vi "DisplayJson.vi"(11 "JSON String In":string="[{\"version\":\"1.0.0\",\"header\":{\"creationDate\":\"2022-06-03T00:00:00\",\"remarks\":\"\",\"serialNumber\":\"98172\",\"productNumber\":\"123021.1804\",\"productType\":\"PAA-9L\",\"pressureType\":2,\"productSeries\":\"9L\",\"compensatedTemperatureRange\":{\"min\":-10.0,\"max\":80.0,\"unit\":4},\"compensatedPressureRange\":{\"min\":0.0,\"max\":0.35,\"unit\":3},\"electricSupply\":{\"magnitude\":1.0,\"unit\":18},\"orderNumber\":9990266,\"orderPosition\":3,\"orderTargetDispatchDate\":\"2022-06-02T00:00:00+00:00\",\"customerName\":\"DemoData Inc.\",\"customerNumber\":12345678,\"customerOrderNumber\":\"Cust-9990266-123\",\"customerReferenceNumber\":\"\",\"customerProductT...") -> ()   [LabVIEW 2017] (continued)
\"unit\":4},\"error\":{\"magnitude\":0.10911646,\"unit\":4}}}}}},{\"reference\":\"F_12300_XX_0000098765\",\"environmentTarget\":{\"pressure\":{\"magnitude\":0.11,\"unit\":3},\"temperature\":{\"magnitude\":80.0,\"unit\":4}},\"environment\":{\"pressure\":{\"magnitude\":0.11,\"unit\":3},\"temperature\":{\"magnitude\":79.9513,\"unit\":4},\"supply\":{\"magnitude\":1.0,\"unit\":18}},\"raw\":{\"signal\":{\"magnitude\":34.075381003,\"unit\":22},\"bridgeResistance\":{\"magnitude\":4098.6572078,\"unit\":28}},\"compensated\":{\"mathematicalModels\":{\"MM0123\":{\"pressure\":{\"output\":{\"magnitude\":0.10996,\"unit\":3},\"error\":{\"magnitude\":-0.011442623,\"unit\":7}},\"temperature\":{\"output\":{\"magnitude\":80.0644,\"unit\":4},\"error\":{\"magnitude\":0.11306469,\"unit\":4}}}}}},{\"reference\":\"F_12300_XX_0000098765\",\"environmentTarget\":{\"pressure\":{\"magnitude\":0.19,\"unit\":3},\"temperature\":{\"magnitude\":80.0,\"unit\":4}},\"environment\":{\"pressure\":{\"magnitude\":0.189999,\"unit\":3},\"temperature\":{\"magnitude\":79.9513,\"unit\":4},\"supply\":{\"magnitude\":1.0,\"unit\":18}},\"raw\":{\"signal\":{\"magnitude\":46.277899936,\"unit\":22},\"bridgeResistance\":{\"magnitude\":4094.0695855,\"unit\":28}},\"compensated\":{\"mathematicalModels\":{\"MM0123\":{\"pressure\":{\"output\":{\"magnitude\":0.190002,\"unit\":3},\"error\":{\"magnitude\":0.00090359414,\"unit\":7}},\"temperature\":{\"output\":{\"magnitude\":80.0722,\"unit\":4},\"error\":{\"magnitude\":0.12084368,\"unit\":4}}}}}},{\"reference\":\"F_12300_XX_0000098765\",\"environmentTarget\":{\"pressure\":{\"magnitude\":0.27,\"unit\":3},\"temperature\":{\"magnitude\":80.0,\"unit\":4}},\"environment\":{\"pressure\":{\"magnitude\":0.27,\"unit\":3},\"temperature\":{\"magnitude\":79.9513,\"unit\":4},\"supply\":{\"magnitude\":1.0,\"unit\":18}},\"raw\":{\"signal\":{\"magnitude\":58.449048989,\"unit\":22},\"bridgeResistance\":{\"magnitude\":4089.5073863,\"unit\":28}},\"compensated\":{\"mathematicalModels\":{\"MM0123\":{\"pressure\":{\"output\":{\"magnitude\":0.270033,\"unit\":3},\"error\":{\"magnitude\":0.0095410356,\"unit\":7}},\"temperature\":{\"output\":{\"magnitude\":80.0777,\"unit\":4},\"error\":{\"magnitude\":0.12631932,\"unit\":4}}}}}},{\"reference\":\"F_12300_XX_0000098765\",\"environmentTarget\":{\"pressure\":{\"magnitude\":0.35,\"unit\":3},\"temperature\":{\"magnitude\":80.0,\"unit\":4}},\"environment\":{\"pressure\":{\"magnitude\":0.349991,\"unit\":3},\"temperature\":{\"magnitude\":79.9513,\"unit\":4},\"supply\":{\"magnitude\":1.0,\"unit\":18}},\"raw\":{\"signal\":{\"magnitude\":70.576898184,\"unit\":22},\"bridgeResistance\":{\"magnitude\":4085.0103843,\"unit\":28}},\"compensated\":{\"mathematicalModels\":{\"MM0123\":{\"pressure\":{\"output\":{\"magnitude\":0.349975,\"unit\":3},\"error\":{\"magnitude\":-0.0045630258,\"unit\":7}},\"temperature\":{\"output\":{\"magnitude\":80.084,\"unit\":4},\"error\":{\"magnitude\":0.13265707,\"unit\":4}}}}}}]},{\"version\":\"1.0.0\",\"header\":{\"creationDate\":\"2022-06-03T00:00:00\",\"remarks\":\"\",\"serialNumber\":\"98120\",\"productNumber\":\"123021.1804\",\"productType\":\"PAA-9L\",\"pressureType\":2,\"productSeries\":\"9L\",\"compensatedTemperatureRange\":{\"min\":-10.0,\"max\":80.0,\"unit\":4},\"compensatedPressureRange\":{\"min\":0.0,\"max\":0.35,\"unit\":3},\"electricSupply\":{\"magnitude\":1.0,\"unit\":18},\"orderNumber\":9990266,\"orderPosition\":3,\"orderTargetDispatchDate\":\"2022-06-02T00:00:00+00:00\",\"customerName\":\"DemoData Inc.\",\"customerNumber\":12345678,\"customerOrderNumber\":\"Cust-9990266-123\",\"customerReferenceNumber\":\"\",\"customerProductType\":\"123021-1804 Rev.AA\"},\"compensationMethods\":{\"mathematicalModels\":{\"MM0123\":{\"modelType\":\"MM0123\",\"productNumber\":\"000000.0000\",\"compensatedTemperatureRange\":{\"min\":-10.0,\"max\":80.0,\"unit\":4},\"compensatedPressureRange\":{\"min\":0.0,\"max\":0.35,\"unit\":3},\"electricSupply\":{\"magnitude\":1.0,\"unit\":18},\"parts\":{\"pressure\":{\"inputs\":[\"Sig\",\"R\"],\"output\":\"P\",\"description\":\"P = f(Sig,R)\",\"coefficients\":[[3.80687640842,-0.00383024726793,1.42827172301E-06,-2.38902903502E-10,1.49525310822E-14],[-0.0978417022725,0.000104324759416,-3.89249748451E-08,6.44275711238E-12,-4.00281485262E-16],[-0.000392661762146,4.52316475722E-07,-1.9265072904E-10,3.61496115335E-14,-2.52797959852E-18]]},\"temperature\":{\"inputs\":[\"R\",\"Sig\"],\"output\":\"T\",\"description\":\"T = f(R,Sig)\",\"coefficients\":[[-7952.96201197,-2.02662210439,0.0134421000875],[7.80033862746,0.00330646246975,-1.59232351911E-05],[-0.00293461659049,-1.72390715848E-06,6.89820469355E-09],[5.0021540696E-07,3.72029008192E-10,-1.30570761964E-12],[-3.21770300206E-11,-2.89606535877E-14,9.15121335916E-17]]}}}}},\"measurements\":[{\"reference\":\"F_12300_XX_0000098765\",\"environmentTarget\":{\"pressure\":{\"magnitude\":0.03,\"unit\":3},\"temperature\":{\"magnitude\":-10.0,\"unit\":4}},\"environment\":{\"pressure\":{\"magnitude\":0.0300016,\"unit\":3},\"temperature\":{\"magnitude\":-10.7286,\"unit\":4},\"supply\":{\"magnitude\":1.0,\"unit\":18}},\"raw\":{\"signal\":{\"magnitude\":17.647568183,\"unit\":22},\"bridgeResistance\":{\"magnitude\":3284.2199645,\"unit\":28}},\"compensated\":{\"mathematicalModels\":{\"MM0123\":{\"pressure\":{\"output\":{\"magnitude\":0.0300151,\"unit\":3},\"error\":{\"magnitude\":0.0038534803,\"unit\":7}},\"temperature\":{\"output\":{\"magnitude\":-10.8543,\"unit\":4},\"error\":{\"magnitude\":-0.12565537,\"unit\":4}}}}}},{\"reference\":\"F_12300_XX_0000098765\",\"environmentTarget\":{\"pressure\":{\"magnitude\":0.11,\"unit\":3},\"temperature\":{\"magnitude\":-10.0,\"unit\":4}},\"environment\":{\"pressure\":{\"magnitude\":0.109994,\"unit\":3},\"temperature\":{\"magnitude\":-10.7286,\"unit\":4},\"supply\":{\"magnitude\":1.0,\"unit\":18}},\"raw\":{\"signal\":{\"magnitude\":29.623305989,\"unit\":22},\"bridgeResistance\":{\"magnitude\":3279.6852656,\"unit\":28}},\"compensated\":{\"mathematicalModels\":{\"MM0123\":{\"pressure\":{\"output\":{\"magnitude\":0.10996,\"unit\":3},\"error\":{\"magnitude\":-0.0096543576,\"unit\":7}},\"temperature\":{\"output\":{\"magnitude\":-10.8536,\"unit\":4},\"error\":{\"magnitude\":-0.12492151,\"unit\":4}}}}}},{\"reference\":\"F_12300_XX_0000098765\",\"environmentTarget\":{\"pressure\":{\"magnitude\":0.19,\"unit\":3},\"temperature\":{\"magnitude\":-10.0,\"unit\":4}},\"environment\":{\"pressure\":{\"magnitude\":0.190007,\"unit\":3},\"temperature\":{\"magnitude\":-10.7286,\"unit\":4},\"supply\":{\"magnitude\":1.0,\"unit\":18}},\"raw\":{\"signal\":{\"magnitude\":41.5629955,\"unit\":22},\"bridgeResistance\":{\"magnitude\":3275.2173858,\"unit\":28}},\"compensated\":{\"mathematicalModels\":{\"MM0123\":{\"pressure\":{\"output\":{\"magnitude\":0.190015,\"unit\":3},\"error\":{\"magnitude\":0.0022835569,\"unit\":7}},\"temperature\":{\"output\":{\"magnitude\":-10.8576,\"unit\":4},\"error\":{\"magnitude\":-0.12895315,\"unit\":4}}}}}},{\"reference\":\"F_12300_XX_0000098765\",\"environmentTarget\":{\"pressure\":{\"magnitude\":0.27,\"unit\":3},\"temperature\":{\"magnitude\":-10.0,\"unit\":4}},\"environment\":{\"pressure\":{\"magnitude\":0.270011,\"unit\":3},\"temperature\":{\"magnitude\":-10.7286,\"unit\":4},\"supply\":{\"magnitude\":1.0,\"unit\":18}},\"raw\":{\"signal\":{\"magnitude\":53.446990918,\"unit\":22},\"bridgeResistance\":{\"magnitude\":3270.9221092,\"unit\":28}},\"compensated\":{\"mathematicalModels\":{\"MM0123\":{\"pressure\":{\"output\":{\"magnitude\":0.270044,\"unit\":3},\"error\":{\"magnitude\":0.0095289216,\"unit\":7}},\"temperature\":{\"output\":{\"magnitude\":-10.8518,\"unit\":4},\"error\":{\"magnitude\":-0.12313925,\"unit\":4}}}}}},{\"reference\":\"F_12300_XX_0000098765\",\"environmentTarget\":{\"pressure\":{\"magnitude\":0.35,\"unit\":3},\"temperature\":{\"magnitude\":-10.0,\"unit\":4}},\"environment\":{\"pressure\":{\"magnitude\":0.350004,\"unit\":3},\"temperature\":{\"magnitude\":-10.7286,\"unit\":4},\"supply\":{\"magnitude\":1.0,\"unit\":18}},\"raw\":{\"signal\":{\"magnitude\":65.267069587,\"unit\":22},\"bridgeResistance\":{\"magnitude\":3266.656716,\"unit\":28}},\"compensated\":{\"mathematicalModels\":{\"MM0123\":{\"pressure\":{\"output\":{\"magnitude\":0.349998,\"unit\":3},\"error\":{\"magnitude\":-0.0016541156,\"unit\":7}},\"temperature\":{\"output\":{\"magnitude\":-10.8581,\"unit\":4},\"error\":{\"magnitude\":-0.12948393,\"unit\":4}}}}}},{\"reference\":\"F_12300_XX_0000098765\",\"environmentTarget\":{\"pressure\":{\"magnitude\":0.03,\"unit\":3},\"temperature\":{\"magnitude\":0.0,\"unit\":4}},\"environment\":{\"pressure\":{\"magnitude\":0.0300081,\"unit\":3},\"temperature\":{\"magnitude\":-0.629962,\"unit\":4},\"supply\":{\"magnitude\":1.0,\"unit\":18}},\"raw\":{\"signal\":{\"magnitude\":18.166060326,\"unit\":22},\"bridgeResistance\":{\"magnitude\":3353.9752499,\"unit\":28}},\"compensated\":{\"mathematicalModels\":{\"MM0123\":{\"pressure\":{\"output\":{\"magnitude\":0.030027,\"unit\":3},\"error\":{\"magnitude\":0.0053956345,\"unit\":7}},\"temperature\":{\"output\":{\"magnitude\":-0.756227,\"unit\":4},\"error\":{\"magnitude\":-0.12626536,\"unit\":4}}}}}},{\"reference\":\"F_12300_XX_0000098765\",\"environmentTarget\":{\"pressure\":{\"magnitude\":0.11,\"unit\":3},\"temperature\":{\"magnitude\":0.0,\"unit\":4}},\"environment\":{\"pressure\":{\"magnitude\":0.110003,\"unit\":3},\"temperature\":{\"magnitude\":-0.629962,\"unit\":4},\"supply\":{\"magnitude\":1.0,\"unit\":18}},\"raw\":{\"signal\":{\"magnitude\":30.109259393,\"unit\":22},\"bridgeResistance\":{\"magnitude\":3349.3967264,\"unit\":28}},\"compensated\":{\"mathematicalModels\":{\"MM0123\":{\"pressure\":{\"output\":{\"magnitude\":0.109974,\"unit\":3},\"error\":{\"magnitude\":-0.0081737866,\"unit\":7}},\"temperature\":{\"output\":{\"magnitude\":-0.762387,\"unit\":4},\"error\":{\"magnitude\":-0.13242561,\"unit\":4}}}}}},{\"reference\":\"F_12300_XX_0000098765\",\"environmentTarget\":{\"pressure\":{\"magnitude\":0.19,\"unit\":3},\"temperature\":{\"magnitude\":0.0,\"unit\":4}},\"environment\":{\"pressure\":{\"magnitude\":0.19,\"unit\":3},\"temperature\":{\"magnitude\":-0.629962,\"unit\":4},\"supply\":{\"magnitude\":1.0,\"unit\":18}},\"raw\":{\"signal\":{\"magnitude\":42.013989643,\"unit\":22},\"bridgeResistance\":{\"magnitude\":3344.9475418,\"unit\":28}},\"compensated\":{\"mathematicalModels\":{\"MM0123\":{\"pressure\":{\"output\":{\"magnitude\":0.189997,\"unit\":3},\"error\":{\"magnitude\":-0.00074399073,\"unit\":7}},\"temperature\":{\"output\":{\"magnitude\":-0.763716,\"unit\":4},\"error\":{\"magnitude\":-0.13375452,\"unit\":4}}}}}},{\"reference\":\"F_12300_XX_0000098765\",\"environmentTarget\":{\"pressure\":{\"magnitude\":0.27,\"unit\":3},\"temperature\":{\"magnitude\":0.0,\"unit\":4}},\"environment\":{\"pressure\":{\"magnitude\":0.270002,\"unit\":3},\"temperature\":{\"magnitude\":-0.629962,\"unit\":4},\"supply\":{\"magnitude\":1.0,\"unit\":18}},\"raw\":{\"signal\":{\"magnitude\":53.868228434,\"unit\":22},\"bridgeResistance\":{\"magnitude\":3340.5943615,\"unit\":28}},\"compensated\":{\"mathematicalModels\":{\"MM0123\":{\"pressure\":{\"output\":{\"magnitude\":0.270018,\"unit\":3},\"error\":{\"magnitude\":0.004524908,\"unit\":7}},\"temperature\":{\"output\":{\"magnitude\":-0.765646,\"unit\":4},\"error\":{\"magnitude\":-0.1356837,\"unit\":4}}}}}},{\"reference\":\"F_12300_XX_0000098765\",\"environmentTarget\":{\"pressure\":{\"magnitude\":0.35,\"unit\":3},\"temperature\":{\"magnitude\":0.0,\"unit\":4}},\"environment\":{\"pressure\":{\"magnitude\":0.349999,\"unit\":3},\"temperature\":{\"magnitude\":-0.629962,\"unit\":4},\"supply\":{\"magnitude\":1.0,\"unit\":18}},\"raw\":{\"signal\":{\"magnitude\":65.662121594,\"unit\":22},\"bridgeResistance\":{\"magnitude\":3336.3273067,\"unit\":28}},\"compensated\":{\"mathematicalModels\":{\"MM0123\":{\"pressure\":{\"output\":{\"magnitude\":0.349969,\"unit\":3},\"error\":{\"magnitude\":-0.0084390485,\"unit\":7}},\"temperature\":{\"output\":{\"magnitude\":-0.770185,\"unit\":4},\"error\":{\"magnitude\":-0.14022289,\"unit\":4}}}}}},{\"reference\":\"F_12300_XX_0000098765\",\"environmentTarget\":{\"pressure\":{\"magnitude\":0.03,\"unit\":3},\"temperature\":{\"magnitude\":20.0,\"unit\":4}},\"environment\":{\"pressure\":{\"magnitude\":0.0300042,\"unit\":3},\"temperature\":{\"magnitude\":19.5509,\"unit\":4},\"supply\":{\"magnitude\":1.0,\"unit\":18}},\"raw\":{\"signal\":{\"magnitude\":19.250087303,\"unit\":22},\"bridgeResistance\":{\"magnitude\":3510.6414258,\"unit\":28}},\"compensated\":{\"mathematicalModels\":{\"MM0123\":{\"pressure\":{\"output\":{\"magnitude\":0.0300123,\"unit\":3},\"error\":{\"magnitude\":0.0023081439,\"unit\":7}},\"temperature\":{\"output\":{\"magnitude\":19.5418,\"unit\":4},\"error\":{\"magnitude\":-0.0090331179,\"unit\":4}}}}}},{\"reference\":\"F_12300_XX_0000098765\",\"environmentTarget\":{\"pressure\":{\"magnitude\":0.11,\"unit\":3},\"temperature\":{\"magnitude\":20.0,\"unit\":4}},\"environment\":{\"pressure\":{\"magnitude\":0.109998,\"unit\":3},\"temperature\":{\"magnitude\":19.5509,\"unit\":4},\"supply\":{\"magnitude\":1.0,\"unit\":18}},\"raw\":{\"signal\":{\"magnitude\":31.186444983,\"unit\":22},\"bridgeResistance\":{\"magnitude\":3506.082338,\"unit\":28}},\"compensated\":{\"mathematicalModels\":{\"MM0123\":{\"pressure\":{\"output\":{\"magnitude\":0.10997,\"unit\":3},\"error\":{\"magnitude\":-0.0078955543,\"unit\":7}},\"temperature\":{\"output\":{\"magnitude\":19.5383,\"unit\":4},\"error\":{\"magnitude\":-0.012599029,\"unit\":4}}}}}},{\"reference\":\"F_12300_XX_0000098765\",\"environmentTarget\":{\"pressure\":{\"magnitude\":0.19,\"unit\":3},\"temperature\":{\"magnitude\":20.0,\"unit\":4}},\"environment\":{\"pressure\":{\"magnitude\":0.190004,\"unit\":3},\"temperature\":{\"magnitude\":19.5509,\"unit\":4},\"supply\":{\"magnitude\":1.0,\"unit\":18}},\"raw\":{\"signal\":{\"magnitude\":43.090541979,\"unit\":22},\"bridgeResistance\":{\"magnitude\":3501.6259945,\"unit\":28}},\"compensated\":{\"mathematicalModels\":{\"MM0123\":{\"pressure\":{\"output\":{\"magnitude\":0.190012,\"unit\":3},\"error\":{\"magnitude\":0.0022122903,\"unit\":7}},\"temperature\":{\"output\":{\"magnitude\":19.5373,\"unit\":4},\"error\":{\"magnitude\":-0.013537079,\"unit\":4}}}}}},{\"reference\":\"F_12300_XX_0000098765\",\"environmentTarget\":{\"pressure\":{\"magnitude\":0.27,\"unit\":3},\"temperature\":{\"magnitude\":20.0,\"unit\":4}},\"environment\":{\"pressure\":{\"magnitude\":0.26999,\"unit\":3},\"temperature\":{\"magnitude\":19.5509,\"unit\":4},\"supply\":{\"magnitude\":1.0,\"unit\":18}},\"raw\":{\"signal\":{\"magnitude\":54.94545419,\"unit\":22},\"bridgeResistance\":{\"magnitude\":3497.2268392,\"unit\":28}},\"compensated\":{\"mathematicalModels\":{\"MM0123\":{\"pressure\":{\"output\":{\"magnitude\":0.270026,\"unit\":3},\"error\":{\"magnitude\":0.010179711,\"unit\":7}},\"temperature\":{\"output\":{\"magnitude\":19.5326,\"unit\":4},\"error\":{\"magnitude\":-0.018257104,\"unit\":4}}}}}},{\"reference\":\"F_12300_XX_0000098765\",\"environmentTarget\":{\"pressure\":{\"magnitude\":0.35,\"unit\":3},\"temperature\":{\"magnitude\":20.0,\"unit\":4}},\"environment\":{\"pressure\":{\"magnitude\":0.350004,\"unit\":3},\"temperature\":{\"magnitude\":19.5509,\"unit\":4},\"supply\":{\"magnitude\":1.0,\"unit\":18}},\"raw\":{\"signal\":{\"magnitude\":66.750905832,\"unit\":22},\"bridgeResistance\":{\"magnitude\":3492.9257957,\"unit\":28}},\"compensated\":{\"mathematicalModels\":{\"MM0123\":{\"pressure\":{\"output\":{\"magnitude\":0.350008,\"unit\":3},\"error\":{\"magnitude\":0.0011472352,\"unit\":7}},\"temperature\":{\"output\":{\"magnitude\":19.5289,\"unit\":4},\"error\":{\"magnitude\":-0.021937225,\"unit\":4}}}}}},{\"reference\":\"F_12300_XX_0000098765\",\"environmentTarget\":{\"pressure\":{\"magnitude\":0.03,\"unit\":3},\"temperature\":{\"magnitude\":40.0,\"unit\":4}},\"environment\":{\"pressure\":{\"magnitude\":0.0300015,\"unit\":3},\"temperature\":{\"magnitude\":39.7284,\"unit\":4},\"supply\":{\"magnitude\":1.0,\"unit\":18}},\"raw\":{\"signal\":{\"magnitude\":20.420124301,\"unit\":22},\"bridgeResistance\":{\"magnitude\":3686.7238099,\"unit\":28}},\"compensated\":{\"mathematicalModels\":{\"MM0123\":{\"pressure\":{\"output\":{\"magnitude\":0.0300187,\"unit\":3},\"error\":{\"magnitude\":0.0049274867,\"unit\":7}},\"temperature\":{\"output\":{\"magnitude\":39.7226,\"unit\":4},\"error\":{\"magnitude\":-0.0057734048,\"unit\":4}}}}}},{\"reference\":\"F_12300_XX_0000098765\",\"environmentTarget\":{\"pressure\":{\"magnitude\":0.11,\"unit\":3},\"temperature\":{\"magnitude\":40.0,\"unit\":4}},\"environment\":{\"pressure\":{\"magnitude\":0.11,\"unit\":3},\"temperature\":{\"magnitude\":39.7284,\"unit\":4},\"supply\":{\"magnitude\":1.0,\"unit\":18}},\"raw\":{\"signal\":{\"magnitude\":32.411386537,\"unit\":22},\"bridgeResistance\":{\"magnitude\":3682.1564541,\"unit\":28}},\"compensated\":{\"mathematicalModels\":{\"MM0123\":{\"pressure\":{\"output\":{\"magnitude\":0.109971,\"unit\":3},\"error\":{\"magnitude\":-0.0081534102,\"unit\":7}},\"temperature\":{\"output\":{\"magnitude\":39.7218,\"unit\":4},\"error\":{\"magnitude\":-0.0066173733,\"unit\":4}}}}}},{\"reference\":\"F_12300_XX_0000098765\",\"environmentTarget\":{\"pressure\":{\"magnitude\":0.19,\"unit\":3},\"temperature\":{\"magnitude\":40.0,\"unit\":4}},\"environment\":{\"pressure\":{\"magnitude\":0.190005,\"unit\":3},\"temperature\":{\"magnitude\":39.7284,\"unit\":4},\"supply\":{\"magnitude\":1.0,\"unit\":18}},\"raw\":{\"signal\":{\"magnitude\":44.374338351,\"unit\":22},\"bridgeResistance\":{\"magnitude\":3677.629143,\"unit\":28}},\"compensated\":{\"mathematicalModels\":{\"MM0123\":{\"pressure\":{\"output\":{\"magnitude\":0.190003,\"unit\":3},\"error\":{\"magnitude\":-0.00064036846,\"unit\":7}},\"temperature\":{\"output\":{\"magnitude\":39.7177,\"unit\":4},\"error\":{\"magnitude\":-0.010704785,\"unit\":4}}}}}},{\"reference\":\"F_12300_XX_0000098765\",\"environmentTarget\":{\"pressure\":{\"magnitude\":0.27,\"unit\":3},\"temperature\":{\"magnitude\":40.0,\"unit\":4}},\"environment\":{\"pressure\":{\"magnitude\":0.269997,\"unit\":3},\"temperature\":{\"magnitude\":39.7284,\"unit\":4},\"supply\":{\"magnitude\":1.0,\"unit\":18}},\"raw\":{\"signal\":{\"magnitude\":56.294892967,\"unit\":22},\"bridgeResistance\":{\"magnitude\":3673.2124389,\"unit\":28}},\"compensated\":{\"mathematicalModels\":{\"MM0123\":{\"pressure\":{\"output\":{\"magnitude\":0.270015,\"unit\":3},\"error\":{\"magnitude\":0.0052162958,\"unit\":7}},\"temperature\":{\"output\":{\"magnitude\":39.7174,\"unit\":4},\"error\":{\"magnitude\":-0.010996395,\"unit\":4}}}}}},{\"reference\":\"F_12300_XX_0000098765\",\"environmentTarget\":{\"pressure\":{\"magnitude\":0.35,\"unit\":3},\"temperature\":{\"magnitude\":40.0,\"unit\":4}},\"environment\":{\"pressure\":{\"magnitude\":0.350001,\"unit\":3},\"temperature\":{\"magnitude\":39.7284,\"unit\":4},\"supply\":{\"magnitude\":1.0,\"unit\":18}},\"raw\":{\"signal\":{\"magnitude\":68.167917174,\"unit\":22},\"bridgeResistance\":{\"magnitude\":3668.869247,\"unit\":28}},\"compensated\":{\"mathematicalModels\":{\"MM0123\":{\"pressure\":{\"output\":{\"magnitude\":0.349976,\"unit\":3},\"error\":{\"magnitude\":-0.007225637,\"unit\":7}},\"temperature\":{\"output\":{\"magnitude\":39.7166,\"unit\":4},\"error\":{\"magnitude\":-0.01179225,\"unit\":4}}}}}},{\"reference\":\"F_12300_XX_0000098765\",\"environmentTarget\":{\"pressure\":{\"magnitude\":0.03,\"unit\":3},\"temperature\":{\"magnitude\":60.0,\"unit\":4}},\"environment\":{\"pressure\":{\"magnitude\":0.029997,\"unit\":3},\"temperature\":{\"magnitude\":59.8651,\"unit\":4},\"supply\":{\"magnitude\":1.0,\"unit\":18}},\"raw\":{\"signal\":{\"magnitude\":21.708177229,\"unit\":22},\"bridgeResistance\":{\"magnitude\":3879.4432643,\"unit\":28}},\"compensated\":{\"mathematicalModels\":{\"MM0123\":{\"pressure\":{\"output\":{\"magnitude\":0.0300116,\"unit\":3},\"error\":{\"magnitude\":0.0041652623,\"unit\":7}},\"temperature\":{\"output\":{\"magnitude\":59.9377,\"unit\":4},\"error\":{\"magnitude\":0.072550935,\"unit\":4}}}}}},{\"reference\":\"F_12300_XX_0000098765\",\"environmentTarget\":{\"pressure\":{\"magnitude\":0.11,\"unit\":3},\"temperature\":{\"magnitude\":60.0,\"unit\":4}},\"environment\":{\"pressure\":{\"magnitude\":0.110005,\"unit\":3},\"temperature\":{\"magnitude\":59.8651,\"unit\":4},\"supply\":{\"magnitude\":1.0,\"unit\":18}},\"raw\":{\"signal\":{\"magnitude\":33.797708383,\"unit\":22},\"bridgeResistance\":{\"magnitude\":3874.809144,\"unit\":28}},\"compensated\":{\"mathematicalModels\":{\"MM0123\":{\"pressure\":{\"output\":{\"magnitude\":0.109973,\"unit\":3},\"error\":{\"magnitude\":-0.0090400862,\"unit\":7}},\"temperature\":{\"output\":{\"magnitude\":59.9392,\"unit\":4},\"error\":{\"magnitude\":0.074114492,\"unit\":4}}}}}},{\"reference\":\"F_12300_XX_0000098765\",\"environmentTarget\":{\"pressure\":{\"magnitude\":0.19,\"unit\":3},\"temperature\":{\"magnitude\":60.0,\"unit\":4}},\"environment\":{\"pressure\":{\"magnitude\":0.190006,\"unit\":3},\"temperature\":{\"magnitude\":59.8651,\"unit\":4},\"supply\":{\"magnitude\":1.0,\"unit\":18}},\"raw\":{\"signal\":{\"magnitude\":45.862942853,\"unit\":22},\"bridgeResistance\":{\"magnitude\":3870.2562199,\"unit\":28}},\"compensated\":{\"mathematicalModels\":{\"MM0123\":{\"pressure\":{\"output\":{\"magnitude\":0.19001,\"unit\":3},\"error\":{\"magnitude\":0.0011682051,\"unit\":7}},\"temperature\":{\"output\":{\"magnitude\":59.9427,\"unit\":4},\"error\":{\"magnitude\":0.077596604,\"unit\":4}}}}}},{\"reference\":\"F_12300_XX_0000098765\",\"environmentTarget\":{\"pressure\":{\"magnitude\":0.27,\"unit\":3},\"temperature\":{\"magnitude\":60.0,\"unit\":4}},\"environment\":{\"pressure\":{\"magnitude\":0.270009,\"unit\":3},\"temperature\":{\"magnitude\":59.8651,\"unit\":4},\"supply\":{\"magnitude\":1.0,\"unit\":18}},\"raw\":{\"signal\":{\"magnitude\":57.891186272,\"unit\":22},\"bridgeResistance\":{\"magnitude\":3865.740431,\"unit\":28}},\"compensated\":{\"mathematicalModels\":{\"MM0123\":{\"pressure\":{\"output\":{\"magnitude\":0.27004,\"unit\":3},\"error\":{\"magnitude\":0.0089952809,\"unit\":7}},\"temperature\":{\"output\":{\"magnitude\":59.9432,\"unit\":4},\"error\":{\"magnitude\":0.078035411,\"unit\":4}}}}}},{\"reference\":\"F_12300_XX_0000098765\",\"environmentTarget\":{\"pressure\":{\"magnitude\":0.35,\"unit\":3},\"temperature\":{\"magnitude\":60.0,\"unit\":4}},\"environment\":{\"pressure\":{\"magnitude\":0.349994,\"unit\":3},\"temperature\":{\"magnitude\":59.8651,\"unit\":4},\"supply\":{\"magnitude\":1.0,\"unit\":18}},\"raw\":{\"signal\":{\"magnitude\":69.871054861,\"unit\":22},\"bridgeResistance\":{\"magnitude\":3861.3226917,\"unit\":28}},\"compensated\":{\"mathematicalModels\":{\"MM0123\":{\"pressure\":{\"output\":{\"magnitude\":0.349984,\"unit\":3},\"error\":{\"magnitude\":-0.0028963517,\"unit\":7}},\"temperature\":{\"output\":{\"magnitude\":59.9463,\"unit\":4},\"error\":{\"magnitude\":0.081135385,\"unit\":4}}}}}},{\"reference\":\"F_12300_XX_0000098765\",\"environmentTarget\":{\"pressure\":{\"magnitude\":0.03,\"unit\":3},\"temperature\":{\"magnitude\":80.0,\"unit\":4}},\"environment\":{\"pressure\":{\"magnitude\":0.0299997,\"unit\":3},\"temperature\":{\"magnitude\":79.9513,\"unit\":4},\"supply\":{\"magnitude\":1.0,\"unit\":18}},\"raw\":{\"signal\":{\"magnitude\":23.157485274,\"unit\":22},\"bridgeResistance\":{\"magnitude\":4087.1289356,\"unit\":28}},\"compensated\":{\"mathematicalModels\":{\"MM0123\":{\"pressure\":{\"output\":{\"magnitude\":0.0300165,\"unit\":3},\"error\":{\"magnitude\":0.0048100854,\"unit\":7}},\"temperature\":{\"output\":{\"magnitude\":80.0622,\"unit\":4},\"error\":{\"magnitude\":0.11086344,\"unit\":4}}}}}},{\"reference\":\"F_12300_XX_0000098765\",\"environmentTarget\":{\"pressure\":{\"magnitude\":0.11,\"unit\":3},\"temperature\":{\"magnitude\":80.0,\"unit\":4}},\"environment\":{\"pressure\":{\"magnitude\":0.110003,\"unit\":3},\"temperature\":{\"magnitude\":79.9513,\"unit\":4},\"supply\":{\"magnitude\":1.0,\"unit\":18}},\"raw\":{\"signal\":{\"magnitude\":35.370411541,\"unit\":22},\"bridgeResistance\":{\"magnitude\":4082.408777,\"unit\":28}},\"compensated\":{\"mathematicalModels\":{\"MM0123\":{\"pressure\":{\"output\":{\"magnitude\":0.109963,\"unit\":3},\"error\":{\"magnitude\":-0.011389484,\"unit\":7}},\"temperature\":{\"output\":{\"magnitude\":80.0646,\"unit\":4},\"error\":{\"magnitude\":0.11330273,\"unit\":4}}}}}},{\"reference\":\"F_12300_XX_0000098765\",\"environmentTarget\":{\"pressure\":{\"magnitude\":0.19,\"unit\":3},\"temperature\":{\"magnitude\":80.0,\"unit\":4}},\"environment\":{\"pressure\":{\"magnitude\":0.189998,\"unit\":3},\"temperature\":{\"magnitude\":79.9513,\"unit\":4},\"supply\":{\"magnitude\":1.0,\"unit\":18}},\"raw\":{\"signal\":{\"magnitude\":47.568169907,\"unit\":22},\"bridgeResistance\":{\"magnitude\":4077.8130815,\"unit\":28}},\"compensated\":{\"mathematicalModels\":{\"MM0123\":{\"pressure\":{\"output\":{\"magnitude\":0.190003,\"unit\":3},\"error\":{\"magnitude\":0.0014154094,\"unit\":7}},\"temperature\":{\"output\":{\"magnitude\":80.0743,\"unit\":4},\"error\":{\"magnitude\":0.12297589,\"unit\":4}}}}}},{\"reference\":\"F_12300_XX_0000098765\",\"environmentTarget\":{\"pressure\":{\"magnitude\":0.27,\"unit\":3},\"temperature\":{\"magnitude\":80.0,\"unit\":4}},\"environment\":{\"pressure\":{\"magnitude\":0.270002,\"unit\":3},\"temperature\":{\"magnitude\":79.9513,\"unit\":4},\"supply\":{\"magnitude\":1.0,\"unit\":18}},\"raw\":{\"signal\":{\"magnitude\":59.733957012,\"unit\":22},\"bridgeResistance\":{\"magnitude\":4073.2290559,\"unit\":28}},\"compensated\":{\"mathematicalModels\":{\"MM0123\":{\"pressure\":{\"output\":{\"magnitude\":0.270035,\"unit\":3},\"error\":{\"magnitude\":0.0093336091,\"unit\":7}},\"temperature\":{\"output\":{\"magnitude\":80.0802,\"unit\":4},\"error\":{\"magnitude\":0.12890837,\"unit\":4}}}}}},{\"reference\":\"F_12300_XX_0000098765\",\"environmentTarget\":{\"pressure\":{\"magnitude\":0.35,\"unit\":3},\"temperature\":{\"magnitude\":80.0,\"unit\":4}},\"environment\":{\"pressure\":{\"magnitude\":0.349992,\"unit\":3},\"temperature\":{\"magnitude\":79.9513,\"unit\":4},\"supply\":{\"magnitude\":1.0,\"unit\":18}},\"raw\":{\"signal\":{\"magnitude\":71.855409902,\"unit\":22},\"bridgeResistance\":{\"magnitude\":4068.7002457,\"unit\":28}},\"compensated\":{\"mathematicalModels\":{\"MM0123\":{\"pressure\":{\"output\":{\"magnitude\":0.349977,\"unit\":3},\"error\":{\"magnitude\":-0.0043503903,\"unit\":7}},\"temperature\":{\"output\":{\"magnitude\":80.0856,\"unit\":4},\"error\":{\"magnitude\":0.1342656,\"unit\":4}}}}}}]},{\"version\":\"1.0.0\",\"header\":{\"creationDate\":\"2022-06-03T00:00:00\",\"remarks\":\"\",\"serialNumber\":\"98100\",\"productNumber\":\"123021.1804\",\"productType\":\"PAA-9L\",\"pressureType\":2,\"productSeries\":\"9L\",\"compensatedTemperatureRange\":{\"min\":-10.0,\"max\":80.0,\"unit\":4},\"compensatedPressureRange\":{\"min\":0.0,\"max\":0.35,\"unit\":3},\"electricSupply\":{\"magnitude\":1.0,\"unit\":18},\"orderNumber\":9990266,\"orderPosition\":3,\"orderTargetDispatchDate\":\"2022-06-02T00:00:00+00:00\",\"customerName\":\"DemoData Inc.\",\"customerNumber\":12345678,\"customerOrderNumber\":\"Cust-9990266-123\",\"customerReferenceNumber\":\"\",\"customerProductType\":\"123021-1804 Rev.AA\"},\"compensationMethods\":{\"mathematicalModels\":{\"MM0123\":{\"modelType\":\"MM0123\",\"productNumber\":\"000000.0000\",\"compensatedTemperatureRange\":{\"min\":-10.0,\"max\":80.0,\"unit\":4},\"compensatedPressureRange\":{\"min\":0.0,\"max\":0.35,\"unit\":3},\"electricSupply\":{\"magnitude\":1.0,\"unit\":18},\"parts\":{\"pressure\":{\"inputs\":[\"Sig\",\"R\"],\"output\":\"P\",\"description\":\"P = f(Sig,R)\",\"coefficients\":[[4.19409509975,-0.0042927971195,1.63472763544E-06,-2.78670685584E-10,1.77945226213E-14],[-0.129538997916,0.000139406977521,-5.33003739123E-08,9.05066087175E-12,-5.77136978351E-16],[-9.70678436406E-05,1.33776620244E-07,-6.42632595062E-11,1.32152549916E-14,-9.96099299559E-19]]},\"temperature\":{\"inputs\":[\"R\",\"Sig\"],\"output\":\"T\",\"description\":\"T = f(R,Sig)\",\"coefficients\":[[-7989.05435389,-3.13251075163,0.0277395225294],[7.90360678785,0.00468634525679,-3.33046732959E-05],[-0.00299951378574,-2.36480738727E-06,1.47300400333E-08],[5.15727935192E-07,5.03173898294E-10,-2.85814202877E-12],[-3.34625849699E-11,-3.89321469435E-14,2.05859762351E-16]]}}}}},\"measurements\":[{\"reference\":\"F_12300_XX_0000098765\",\"environmentTarget\":{\"pressure\":{\"magnitude\":0.03,\"unit\":3},\"temperature\":{\"magnitude\":-10.0,\"unit\":4}},\"environment\":{\"pressure\":{\"magnitude\":0.0300061,\"unit\":3},\"temperature\":{\"magnitude\":-10.7286,\"unit\":4},\"supply\":{\"magnitude\":1.0,\"unit\":18}},\"raw\":{\"signal\":{\"magnitude\":14.895369777,\"unit\":22},\"bridgeResistance\":{\"magnitude\":3265.1743906,\"unit\":28}},\"compensated\":{\"mathematicalModels\":{\"MM0123\":{\"pressure\":{\"output\":{\"magnitude\":0.0300152,\"unit\":3},\"error\":{\"magnitude\":0.0026060565,\"unit\":7}},\"temperature\":{\"output\":{\"magnitude\":-10.8355,\"unit\":4},\"error\":{\"magnitude\":-0.10691075,\"unit\":4}}}}}},{\"reference\":\"F_12300_XX_0000098765\",\"environmentTarget\":{\"pressure\":{\"magnitude\":0.11,\"unit\":3},\"temperature\":{\"magnitude\":-10.0,\"unit\":4}},\"environment\":{\"pressure\":{\"magnitude\":0.109996,\"unit\":3},\"temperature\":{\"magnitude\":-10.7286,\"unit\":4},\"supply\":{\"magnitude\":1.0,\"unit\":18}},\"raw\":{\"signal\":{\"magnitude\":26.426186716,\"unit\":22},\"bridgeResistance\":{\"magnitude\":3260.7815362,\"unit\":28}},\"compensated\":{\"mathematicalModels\":{\"MM0123\":{\"pressure\":{\"output\":{\"magnitude\":0.109966,\"unit\":3},\"error\":{\"magnitude\":-0.0086948419,\"unit\":7}},\"temperature\":{\"output\":{\"magnitude\":-10.838,\"unit\":4},\"error\":{\"magnitude\":-0.10932973,\"unit\":4}}}}}},{\"reference\":\"F_12300_XX_0000098765\",\"environmentTarget\":{\"pressure\":{\"magnitude\":0.19,\"unit\":3},\"temperature\":{\"magnitude\":-10.0,\"unit\":4}},\"environment\":{\"pressure\":{\"magnitude\":0.190006,\"unit\":3},\"temperature\":{\"magnitude\":-10.7286,\"unit\":4},\"supply\":{\"magnitude\":1.0,\"unit\":18}},\"raw\":{\"signal\":{\"magnitude\":37.922301195,\"unit\":22},\"bridgeResistance\":{\"magnitude\":3256.505355,\"unit\":28}},\"compensated\":{\"mathematicalModels\":{\"MM0123\":{\"pressure\":{\"output\":{\"magnitude\":0.190013,\"unit\":3},\"error\":{\"magnitude\":0.0019918704,\"unit\":7}},\"temperature\":{\"output\":{\"magnitude\":-10.8378,\"unit\":4},\"error\":{\"magnitude\":-0.10919276,\"unit\":4}}}}}},{\"reference\":\"F_12300_XX_0000098765\",\"environmentTarget\":{\"pressure\":{\"magnitude\":0.27,\"unit\":3},\"temperature\":{\"magnitude\":-10.0,\"unit\":4}},\"environment\":{\"pressure\":{\"magnitude\":0.270002,\"unit\":3},\"temperature\":{\"magnitude\":-10.7286,\"unit\":4},\"supply\":{\"magnitude\":1.0,\"unit\":18}},\"raw\":{\"signal\":{\"magnitude\":49.365591325,\"unit\":22},\"bridgeResistance\":{\"magnitude\":3252.3738774,\"unit\":28}},\"compensated\":{\"mathematicalModels\":{\"MM0123\":{\"pressure\":{\"output\":{\"magnitude\":0.270032,\"unit\":3},\"error\":{\"magnitude\":0.0087094338,\"unit\":7}},\"temperature\":{\"output\":{\"magnitude\":-10.8322,\"unit\":4},\"error\":{\"magnitude\":-0.10355194,\"unit\":4}}}}}},{\"reference\":\"F_12300_XX_0000098765\",\"environmentTarget\":{\"pressure\":{\"magnitude\":0.35,\"unit\":3},\"temperature\":{\"magnitude\":-10.0,\"unit\":4}},\"environment\":{\"pressure\":{\"magnitude\":0.350002,\"unit\":3},\"temperature\":{\"magnitude\":-10.7286,\"unit\":4},\"supply\":{\"magnitude\":1.0,\"unit\":18}},\"raw\":{\"signal\":{\"magnitude\":60.751582832,\"unit\":22},\"bridgeResistance\":{\"magnitude\":3248.2650619,\"unit\":28}},\"compensated\":{\"mathematicalModels\":{\"MM0123\":{\"pressure\":{\"output\":{\"magnitude\":0.349998,\"unit\":3},\"error\":{\"magnitude\":-0.0012594457,\"unit\":7}},\"temperature\":{\"output\":{\"magnitude\":-10.8398,\"unit\":4},\"error\":{\"magnitude\":-0.11220789,\"unit\":4}}}}}},{\"reference\":\"F_12300_XX_0000098765\",\"environmentTarget\":{\"pressure\":{\"magnitude\":0.03,\"unit\":3},\"temperature\":{\"magnitude\":0.0,\"unit\":4}},\"environment\":{\"pressure\":{\"magnitude\":0.0299993,\"unit\":3},\"temperature\":{\"magnitude\":-0.629962,\"unit\":4},\"supply\":{\"magnitude\":1.0,\"unit\":18}},\"raw\":{\"signal\":{\"magnitude\":15.349169703,\"unit\":22},\"bridgeResistance\":{\"magnitude\":3334.7827897,\"unit\":28}},\"compensated\":{\"mathematicalModels\":{\"MM0123\":{\"pressure\":{\"output\":{\"magnitude\":0.0300176,\"unit\":3},\"error\":{\"magnitude\":0.0052417534,\"unit\":7}},\"temperature\":{\"output\":{\"magnitude\":-0.744207,\"unit\":4},\"error\":{\"magnitude\":-0.11424476,\"unit\":4}}}}}},{\"reference\":\"F_12300_XX_0000098765\",\"environmentTarget\":{\"pressure\":{\"magnitude\":0.11,\"unit\":3},\"temperature\":{\"magnitude\":0.0,\"unit\":4}},\"environment\":{\"pressure\":{\"magnitude\":0.110004,\"unit\":3},\"temperature\":{\"magnitude\":-0.629962,\"unit\":4},\"supply\":{\"magnitude\":1.0,\"unit\":18}},\"raw\":{\"signal\":{\"magnitude\":26.847803696,\"unit\":22},\"bridgeResistance\":{\"magnitude\":3330.374856,\"unit\":28}},\"compensated\":{\"mathematicalModels\":{\"MM0123\":{\"pressure\":{\"output\":{\"magnitude\":0.109977,\"unit\":3},\"error\":{\"magnitude\":-0.007734829,\"unit\":7}},\"temperature\":{\"output\":{\"magnitude\":-0.750308,\"unit\":4},\"error\":{\"magnitude\":-0.12034574,\"unit\":4}}}}}},{\"reference\":\"F_12300_XX_0000098765\",\"environmentTarget\":{\"pressure\":{\"magnitude\":0.19,\"unit\":3},\"temperature\":{\"magnitude\":0.0,\"unit\":4}},\"environment\":{\"pressure\":{\"magnitude\":0.190003,\"unit\":3},\"temperature\":{\"magnitude\":-0.629962,\"unit\":4},\"supply\":{\"magnitude\":1.0,\"unit\":18}},\"raw\":{\"signal\":{\"magnitude\":38.309752318,\"unit\":22},\"bridgeResistance\":{\"magnitude\":3326.1087625,\"unit\":28}},\"compensated\":{\"mathematicalModels\":{\"MM0123\":{\"pressure\":{\"output\":{\"magnitude\":0.190001,\"unit\":3},\"error\":{\"magnitude\":-0.00052968161,\"unit\":7}},\"temperature\":{\"output\":{\"magnitude\":-0.749568,\"unit\":4},\"error\":{\"magnitude\":-0.119606,\"unit\":4}}}}}},{\"reference\":\"F_12300_XX_0000098765\",\"environmentTarget\":{\"pressure\":{\"magnitude\":0.27,\"unit\":3},\"temperature\":{\"magnitude\":0.0,\"unit\":4}},\"environment\":{\"pressure\":{\"magnitude\":0.269995,\"unit\":3},\"temperature\":{\"magnitude\":-0.629962,\"unit\":4},\"supply\":{\"magnitude\":1.0,\"unit\":18}},\"raw\":{\"signal\":{\"magnitude\":49.722623024,\"unit\":22},\"bridgeResistance\":{\"magnitude\":3321.8949754,\"unit\":28}},\"compensated\":{\"mathematicalModels\":{\"MM0123\":{\"pressure\":{\"output\":{\"magnitude\":0.270009,\"unit\":3},\"error\":{\"magnitude\":0.0040269531,\"unit\":7}},\"temperature\":{\"output\":{\"magnitude\":-0.756726,\"unit\":4},\"error\":{\"magnitude\":-0.12676395,\"unit\":4}}}}}},{\"reference\":\"F_12300_XX_0000098765\",\"environmentTarget\":{\"pressure\":{\"magnitude\":0.35,\"unit\":3},\"temperature\":{\"magnitude\":0.0,\"unit\":4}},\"environment\":{\"pressure\":{\"magnitude\":0.350003,\"unit\":3},\"temperature\":{\"magnitude\":-0.629962,\"unit\":4},\"supply\":{\"magnitude\":1.0,\"unit\":18}},\"raw\":{\"signal\":{\"magnitude\":61.082898649,\"unit\":22},\"bridgeResistance\":{\"magnitude\":3317.8063418,\"unit\":28}},\"compensated\":{\"mathematicalModels\":{\"MM0123\":{\"pressure\":{\"output\":{\"magnitude\":0.349972,\"unit\":3},\"error\":{\"magnitude\":-0.0087683227,\"unit\":7}},\"temperature\":{\"output\":{\"magnitude\":-0.757831,\"unit\":4},\"error\":{\"magnitude\":-0.12786937,\"unit\":4}}}}}},{\"reference\":\"F_12300_XX_0000098765\",\"environmentTarget\":{\"pressure\":{\"magnitude\":0.03,\"unit\":3},\"temperature\":{\"magnitude\":20.0,\"unit\":4}},\"environment\":{\"pressure\":{\"magnitude\":0.030001,\"unit\":3},\"temperature\":{\"magnitude\":19.5509,\"unit\":4},\"supply\":{\"magnitude\":1.0,\"unit\":18}},\"raw\":{\"signal\":{\"magnitude\":16.292017139,\"unit\":22},\"bridgeResistance\":{\"magnitude\":3490.9698559,\"unit\":28}},\"compensated\":{\"mathematicalModels\":{\"MM0123\":{\"pressure\":{\"output\":{\"magnitude\":0.030005,\"unit\":3},\"error\":{\"magnitude\":0.0011562117,\"unit\":7}},\"temperature\":{\"output\":{\"magnitude\":19.5476,\"unit\":4},\"error\":{\"magnitude\":-0.0033148219,\"unit\":4}}}}}},{\"reference\":\"F_12300_XX_0000098765\",\"environmentTarget\":{\"pressure\":{\"magnitude\":0.11,\"unit\":3},\"temperature\":{\"magnitude\":20.0,\"unit\":4}},\"environment\":{\"pressure\":{\"magnitude\":0.109996,\"unit\":3},\"temperature\":{\"magnitude\":19.5509,\"unit\":4},\"supply\":{\"magnitude\":1.0,\"unit\":18}},\"raw\":{\"signal\":{\"magnitude\":27.782760828,\"unit\":22},\"bridgeResistance\":{\"magnitude\":3486.5917045,\"unit\":28}},\"compensated\":{\"mathematicalModels\":{\"MM0123\":{\"pressure\":{\"output\":{\"magnitude\":0.109977,\"unit\":3},\"error\":{\"magnitude\":-0.005352039,\"unit\":7}},\"temperature\":{\"output\":{\"magnitude\":19.5442,\"unit\":4},\"error\":{\"magnitude\":-0.0066289757,\"unit\":4}}}}}},{\"reference\":\"F_12300_XX_0000098765\",\"environmentTarget\":{\"pressure\":{\"magnitude\":0.19,\"unit\":3},\"temperature\":{\"magnitude\":20.0,\"unit\":4}},\"environment\":{\"pressure\":{\"magnitude\":0.190007,\"unit\":3},\"temperature\":{\"magnitude\":19.5509,\"unit\":4},\"supply\":{\"magnitude\":1.0,\"unit\":18}},\"raw\":{\"signal\":{\"magnitude\":39.240813471,\"unit\":22},\"bridgeResistance\":{\"magnitude\":3482.3194068,\"unit\":28}},\"compensated\":{\"mathematicalModels\":{\"MM0123\":{\"pressure\":{\"output\":{\"magnitude\":0.19001,\"unit\":3},\"error\":{\"magnitude\":0.00099470295,\"unit\":7}},\"temperature\":{\"output\":{\"magnitude\":19.5445,\"unit\":4},\"error\":{\"magnitude\":-0.0064222423,\"unit\":4}}}}}},{\"reference\":\"F_12300_XX_0000098765\",\"environmentTarget\":{\"pressure\":{\"magnitude\":0.27,\"unit\":3},\"temperature\":{\"magnitude\":20.0,\"unit\":4}},\"environment\":{\"pressure\":{\"magnitude\":0.269989,\"unit\":3},\"temperature\":{\"magnitude\":19.5509,\"unit\":4},\"supply\":{\"magnitude\":1.0,\"unit\":18}},\"raw\":{\"signal\":{\"magnitude\":50.653633276,\"unit\":22},\"bridgeResistance\":{\"magnitude\":3478.0839316,\"unit\":28}},\"compensated\":{\"mathematicalModels\":{\"MM0123\":{\"pressure\":{\"output\":{\"magnitude\":0.27002,\"unit\":3},\"error\":{\"magnitude\":0.0089934234,\"unit\":7}},\"temperature\":{\"output\":{\"magnitude\":19.5391,\"unit\":4},\"error\":{\"magnitude\":-0.011778731,\"unit\":4}}}}}},{\"reference\":\"F_12300_XX_0000098765\",\"environmentTarget\":{\"pressure\":{\"magnitude\":0.35,\"unit\":3},\"temperature\":{\"magnitude\":20.0,\"unit\":4}},\"environment\":{\"pressure\":{\"magnitude\":0.350004,\"unit\":3},\"temperature\":{\"magnitude\":19.5509,\"unit\":4},\"supply\":{\"magnitude\":1.0,\"unit\":18}},\"raw\":{\"signal\":{\"magnitude\":62.022470062,\"unit\":22},\"bridgeResistance\":{\"magnitude\":3473.9564065,\"unit\":28}},\"compensated\":{\"mathematicalModels\":{\"MM0123\":{\"pressure\":{\"output\":{\"magnitude\":0.350013,\"unit\":3},\"error\":{\"magnitude\":0.0024616358,\"unit\":7}},\"temperature\":{\"output\":{\"magnitude\":19.5367,\"unit\":4},\"error\":{\"magnitude\":-0.014127341,\"unit\":4}}}}}},{\"reference\":\"F_12300_XX_0000098765\",\"environmentTarget\":{\"pressure\":{\"magnitude\":0.03,\"unit\":3},\"temperature\":{\"magnitude\":40.0,\"unit\":4}},\"environment\":{\"pressure\":{\"magnitude\":0.0300048,\"unit\":3},\"temperature\":{\"magnitude\":39.7284,\"unit\":4},\"supply\":{\"magnitude\":1.0,\"unit\":18}},\"raw\":{\"signal\":{\"magnitude\":17.306361954,\"unit\":22},\"bridgeResistance\":{\"magnitude\":3666.0692461,\"unit\":28}},\"compensated\":{\"mathematicalModels\":{\"MM0123\":{\"pressure\":{\"output\":{\"magnitude\":0.0300226,\"unit\":3},\"error\":{\"magnitude\":0.0050741097,\"unit\":7}},\"temperature\":{\"output\":{\"magnitude\":39.7199,\"unit\":4},\"error\":{\"magnitude\":-0.0085435445,
